vi "MarvinReport.vi"(0 "HEADER1":string="BLDC 60A CONTROLLER TEST DATA SHEET", 1 "ATR Or":refnum<vi>, 2 "Steps   pfull":string[][](table)=[["1", "Comm. & Motor Test", "", "", "", " ", ""], ["1.1", "RS232 Comm. + Version", "5.4.8", "-", "-", "", ""], ["1.2", "CAN Comm.", "5.4.8", "-", "-", "0.0.0", "FAIL"], ["1.3", "Motor Direction", "OK", "-", "-", "", ""], [" ", "", "", "", "", "", ""], ["2", "Venable Test", "", "", "", "", ""], ["2.1", "VEnable ON", "1000", "+/-100", "rpm", "", ""], ["2.2", "VEnable OFF", "0", "+/-100", "rpm", "", ""], [" ", "", "", "", "", "", ""], ["3", "Up/Down Blower Test", "", "", "", "", ""], ["3.1", "Up switch", "1000", "+/-100", "rpm", "", ""], ["3.2", "Down switch", "0", "+/-100", "rpm", "", ""], [" ", "", "", "", "", "", ""], ["4", "Resistance Merkava 4 Test", "", "", "", "", ""], ["4.1", "Resistor measure 1 position", "6850", "+/-100", "rpm", "", ""], ["4.2", "Resistor measure 2 position", "8300", "+/-100", "rpm", "", ""], ["4.3", "Resistor measure 3 position", "9200", "+/-100", "rpm", "", ""], [" ", "", "", "", "", "", ""], ["5", "Resistance Merkava 3 Test", "", "", "", "", ""], ["5.1", "Resistor measure 4 position", "6850", "+/-100", "rpm", "", ""], ["5.2", "Resistor measure 5 position", "9000", "+/-100", "rpm", "", ""], ["5.3", "Resistor measure 6 position", "9980", "+/-100", "rpm", "", ""], [" ", "", "", "", "", "", ""], ["6", "Resistance Namer Test", "", "", "", "", ""], ["6.1", "Resistor measure 7 position", "8350", "+/-100", "rpm", "", ""], ["6.2", "Resistor measure 8 position", "8900", "+/-100", "rpm", "", ""], ["6.3", "Resistor measure 9 position", "9450", "+/-100", "rpm", "", ""], [" ", "", "", "", "", "", ""], ["7", "Analog Voltage Test", "", "", "", "", ""], ["7.1", "Analog Cmd 0V (Analog Sts)", "0", "+/-0.2", "V", "", ""], ["7.2", "Analog Cmd 0V (Velocity)", "0", "+/-200", "rpm", "", ""], ["7.3", "Analog Cmd 1V (Analog Sts)", "1", "+/-0.2", "V", "", ""], ["7.4", "Analog Cmd 1V (Velocity)", "0", "+/-200", "rpm", "", ""], ["7.5", "Analog Cmd 2V (Analog Sts)", "2", "+/-0.2", "V", "", ""], ["7.6", "Analog Cmd 2V (Velocity)", "0", "+/-200", "rpm", "", ""], ["7.7", "Analog Cmd 3V (Analog Sts)", "3", "+/-0.2", "V", "", ""], ["7.8", "Analog Cmd 3V (Velocity)", "0", "+/-200", "rpm", "", ""], ["7.9", "Analog Cmd 4V (Analog Sts)", "4", "+/-0.2", "V", "", ""], ["7.10", "Analog Cmd 4V (Velocity)", "", "+/-200", "rpm", "", ""], ["7.11", "Analog Cmd 4.5V (Analog Sts)", "4.5", "+/-0.2", "V", "", ""], ["7.12", "Analog Cmd 4.5V (Velocity)", "", "+/-200", "rpm", "", ""], [" ", "", "", "", "", "", ""], ["8", "Motor Run Test", "", "", "", "", ""], ["8.1", "Motor Temperature before Run", "30", "+/-15", "C", "", ""], ["8.2", "Motor Current after 1 min", "47", "+/-3", "A", "", ""], ["8.3", "Motor Temperature after 20 min", "55", "+/-15", "C", "", ""], ["8.4", "Motor Current after 20 min", "47", "+/-3", "A", "", ""], [" ", "", "", "", "", "", ""], ["9", "Conductivity Test", "", "", "", "", ""], ["9.1", "J56 to CHASIS", "< 2m", "-", "ohms", "", ""], ["9.2", "J57 to CHASIS", "< 2m", "-", "ohms", "", ""], ["9.3", "J58 to CHASIS", "< 2m", "-", "ohms", "", ""], ["", "", "", "", "", "", ""], ["10", "Insulation Resistance Test", "", "", "", "", ""], ["10.1", "J56_A to CHASIS", "> 500k", "-", "ohms", "", ""], ["10.2", "J56_B to CHASIS", "> 500k", "-", "ohms", "", ""], ["10.3", "J56_C to CHASIS", "> 500k", "-", "ohms", "", ""], ["10.4", "J57_A to CHASIS", "> 500k", "-", "ohms", "", ""], ["10.5", "J57_B to CHASIS", "> 500k", "-", "ohms", "", ""], ["", "", "", "", "", "", ""], ["11", "Torque Test", "", "", "", "", ""], ["11.1", "Torque wrench by DIN Standard & ", "-", "-", ".", "", ""], ["11.2", "manufacturer's instructions for nut Torque.", "-", "-", ".", "", ""], ["", "", "", "", "", "", ""], ["12", "Blower Calibration", "", "", "", "", ""], ["12.1", "Motor Speed ", "9980", "+/-100", "rpm", "", ""], ["12.2", "Driver Current ", "47", "+/-3", "A", "", ""], ["", "", "", "", "", "", ""], ["13", "Leak Test", "5", "+/-0.2", "psig", "", ""], [" ", "", "", "", "", "", ""], ["14", "Set Production Parameters", "", "", "", "", ""], ["14.1", "Unit Serial number", "239", "-", "-", "", ""], [" ", "", "", "", "", "", ""]] caption="ATR", 3 "ApprovedBy":string="N_A", 5 "pageNum":i32=3, 6 "InputHeaderArray":string[][](array[string])=[["", "P/N: RD000001 ", "", "Date: 22/11/2018"], ["", "DRIVER S/N: ", "", "Time: 10:13"], ["", "Product Rev.: 2C  ", "", "Tested by: hfg"], ["", "Software Ver.: 5.4.8", "", "Approved by: GIDI"], ["", "Parameters Ver.: 0.4", "", ""], ["", "Tester Software Ver.: V0.0.o", "", ""], ["", "Tester HW Rev.: V0.1", "", ""], ["", "DSP BOARD S/N: ", "", ""], ["", "POWER BOARD S/N: ", "", ""], ["", "", "", ""], ["", "", "", ""], ["", "", "", ""], ["", "", "", ""], ["", "", "", " "]], 7 "FILE NAME":string="ATR__22-Nov-18.docx", 9 "Report Folder":path=path "C:/Users/Joseph/Desktop/KineticsReports/ATR__22-Nov-18.docx", 11 "PN":string="1", 12 "error in (no error)":errorcluster, 13 "REV":string="  Rev-5.4.8") -> (4 "path out":path=path "C:/Users/Joseph/Desktop/KineticsReports/ATR__22-Nov-18.docx", 15 "error out":errorcluster)   [LabVIEW 2017]
uses:
  <vilib>/Utility/miscctls.llb/LVRowAndColumnUnsignedTypeDef.ctl
  <vilib>/Utility/NIReport.llb/Append Image to Report (path wrap).vi
  <vilib>/Utility/NIReport.llb/Append Text Table to Report (wrap).vi
  <vilib>/Utility/NIReport.llb/Append Report Text (str wrap).vi
  <vilib>/Utility/NIReport.llb/NI_report.lvclass
  <vilib>/Utility/NIReport.llb/Word/NI_Word.lvclass
  <vilib>/addons/_office/NI_ReportGenerationToolkit.lvlib
panel:
  out "size(s)":i32[](array[numeric])
  out "error out 2":errorcluster
  out "RefArr":u32[](array[numeric])=[2875195627, 2876244204, 2878341358]
  in  "Tab Control":T1(tab)=enum."PART1 "
  out "ERRORS\nLIST":string="Summery of Results (Fails Only) :  \t1.2  FAIL !"
  out "Steps   p1":string[][](table)=[["1", "Comm. & Motor Test", "", "", "", " ", ""], ["1.1", "RS232 Comm. + Version", "5.4.8", "-", "-", "", ""], ["1.2", "CAN Comm.", "5.4.8", "-", "-", "", ""], ["1.3", "Motor Direction", "OK", "-", "-", "", ""], [" ", "", "", "", "", "", ""], ["2", "Venable Test", "", "", "", "", ""], ["2.1", "VEnable ON", "1000", "+/-100", "rpm", "", ""], ["2.2", "VEnable OFF", "0", "+/-100", "rpm", "", ""], [" ", "", "", "", "", "", ""], ["3", "Up/Down Blower Test", "", "", "", "", ""], ["3.1", "Up switch", "1000", "+/-100", "rpm", "", ""], ["3.2", "Down switch", "0", "+/-100", "rpm", "", ""], [" ", "", "", "", "", "", ""], ["4", "Resistance Merkava 4 Test", "", "", "", "", ""], ["4.1", "Resistor measure 1 position", "6850", "+/-100", "rpm", "", ""], ["4.2", "Resistor measure 2 position", "8300", "+/-100", "rpm", "", ""], ["4.3", "Resistor measure 3 position", "9200", "+/-100", "rpm", "", ""], [" ", "", "", "", "", "", ""], ["5", "Resistance Merkava 3 Test", "", "", "", "", ""], ["5.1", "Resistor measure 4 position", "6850", "+/-100", "rpm", "", ""], ["5.2", "Resistor measure 5 position", "9000", "+/-100", "rpm", "", ""], ["5.3", "Resistor measure 6 position", "9980", "+/-100", "rpm", "", ""], [" ", "", "", "", "", "", ""], ["6", "Resistance Namer Test", "", "", "", "", ""], ["6.1", "Resistor measure 7 position", "8350", "+/-100", "rpm", "", ""], ["6.2", "Resistor measure 8 position", "8900", "+/-100", "rpm", "", ""], ["6.3", "Resistor measure 9 position", "9450", "+/-100", "rpm", "", ""], [" ", "", "", "", "", "", ""], ["7", "Analog Voltage Test", "", "", "", "", ""], ["7.1", "Analog Cmd 0V (Analog Sts)", "0", "+/-0.2", "V", "", ""], ["7.2", "Analog Cmd 0V (Velocity)", "0", "+/-200", "rpm", "", ""], ["7.3", "Analog Cmd 1V (Analog Sts)", "1", "+/-0.2", "V", "", ""], ["7.4", "Analog Cmd 1V (Velocity)", "0", "+/-200", "rpm", "", ""], ["7.5", "Analog Cmd 2V (Analog Sts)", "2", "+/-0.2", "V", "", ""], ["7.6", "Analog Cmd 2V (Velocity)", "0", "+/-200", "rpm", "", ""], ["7.7", "Analog Cmd 3V (Analog Sts)", "3", "+/-0.2", "V", "", ""], ["7.8", "Analog Cmd 3V (Velocity)", "0", "+/-200", "rpm", "", ""], ["7.9", "Analog Cmd 4V (Analog Sts)", "4", "+/-0.2", "V", "", ""], ["7.10", "Analog Cmd 4V (Velocity)", "", "+/-200", "rpm", "", ""], ["7.11", "Analog Cmd 4.5V (Analog Sts)", "4.5", "+/-0.2", "V", "", ""], ["7.12", "Analog Cmd 4.5V (Velocity)", "", "+/-200", "rpm", "", ""], [" ", "", "", "", "", "", ""], ["8", "Motor Run Test", "", "", "", "", ""], ["8.1", "Motor Temperature before Run", "30", "+/-15", "C", "", ""], ["8.2", "Motor Current after 1 min", "47", "+/-3", "A", "", ""], ["8.3", "Motor Temperature after 20 min", "55", "+/-15", "C", "", ""], ["8.4", "Motor Current after 20 min", "47", "+/-3", "A", "", ""], [" ", "", "", "", "", "", ""], ["9", "Conductivity Test", "", "", "", "", ""], ["9.1", "J56 to CHASIS", "< 2m", "-", "ohms", "", ""], ["9.2", "J57 to CHASIS", "< 2m", "-", "ohms", "", ""], ["9.3", "J58 to CHASIS", "< 2m", "-", "ohms", "", ""], ["", "", "", "", "", "", ""], ["10", "Insulation Resistance Test", "", "", "", "", ""], ["10.1", "J56_A to CHASIS", "> 500k", "-", "ohms", "", ""], ["10.2", "J56_B to CHASIS", "> 500k", "-", "ohms", "", ""], ["10.3", "J56_C to CHASIS", "> 500k", "-", "ohms", "", ""], ["10.4", "J57_A to CHASIS", "> 500k", "-", "ohms", "", ""], ["10.5", "J57_B to CHASIS", "> 500k", "-", "ohms", "", ""], ["", "", "", "", "", "", ""], ["11", "Torque Test", "", "", "", "", ""], ["11.1", "Torque wrench by DIN Standard & ", "-", "-", ".", "", ""], ["11.2", "manufacturer's instructions for nut Torque.", "-", "-", ".", "", ""], ["", "", "", "", "", "", ""], ["12", "Blower Calibration", "", "", "", "", ""], ["12.1", "Motor Speed ", "9980", "+/-100", "rpm", "", ""], ["12.2", "Driver Current ", "47", "+/-3", "A", "", ""], ["", "", "", "", "", "", ""], ["13", "Leak Test", "5", "+/-0.2", "psig", "", ""], [" ", "", "", "", "", "", ""], ["14", "Set Production Parameters", "", "", "", "", ""], ["14.1", "Unit Serial number", "239", "-", "-", "", ""], [" ", "", "", "", "", "", ""]] caption="ATR"
  out "Steps   p2":string[][](table)=[["1", "Comm. & Motor Test", "", "", "", " ", ""], ["1.1", "RS232 Comm. + Version", "5.4.8", "-", "-", "", ""], ["1.2", "CAN Comm.", "5.4.8", "-", "-", "0.0.0", "FAIL"], ["1.3", "Motor Direction", "OK", "-", "-", "", ""], [" ", "", "", "", "", "", ""], ["2", "Venable Test", "", "", "", "", ""], ["2.1", "VEnable ON", "1000", "+/-100", "rpm", "", ""], ["2.2", "VEnable OFF", "0", "+/-100", "rpm", "", ""], [" ", "", "", "", "", "", ""], ["3", "Up/Down Blower Test", "", "", "", "", ""], ["3.1", "Up switch", "1000", "+/-100", "rpm", "", ""], ["3.2", "Down switch", "0", "+/-100", "rpm", "", ""], [" ", "", "", "", "", "", ""], ["4", "Resistance Merkava 4 Test", "", "", "", "", ""], ["4.1", "Resistor measure 1 position", "6850", "+/-100", "rpm", "", ""], ["4.2", "Resistor measure 2 position", "8300", "+/-100", "rpm", "", ""], ["4.3", "Resistor measure 3 position", "9200", "+/-100", "rpm", "", ""], [" ", "", "", "", "", "", ""], ["5", "Resistance Merkava 3 Test", "", "", "", "", ""], ["5.1", "Resistor measure 4 position", "6850", "+/-100", "rpm", "", ""], ["5.2", "Resistor measure 5 position", "9000", "+/-100", "rpm", "", ""], ["5.3", "Resistor measure 6 position", "9980", "+/-100", "rpm", "", ""], [" ", "", "", "", "", "", ""], ["6", "Resistance Namer Test", "", "", "", "", ""], ["6.1", "Resistor measure 7 position", "8350", "+/-100", "rpm", "", ""], ["6.2", "Resistor measure 8 position", "8900", "+/-100", "rpm", "", ""], ["6.3", "Resistor measure 9 position", "9450", "+/-100", "rpm", "", ""], [" ", "", "", "", "", "", ""], ["7", "Analog Voltage Test", "", "", "", "", ""], ["7.1", "Analog Cmd 0V (Analog Sts)", "0", "+/-0.2", "V", "", ""], ["7.2", "Analog Cmd 0V (Velocity)", "0", "+/-200", "rpm", "", ""], ["7.3", "Analog Cmd 1V (Analog Sts)", "1", "+/-0.2", "V", "", ""], ["7.4", "Analog Cmd 1V (Velocity)", "0", "+/-200", "rpm", "", ""], ["7.5", "Analog Cmd 2V (Analog Sts)", "2", "+/-0.2", "V", "", ""], ["7.6", "Analog Cmd 2V (Velocity)", "0", "+/-200", "rpm", "", ""], ["7.7", "Analog Cmd 3V (Analog Sts)", "3", "+/-0.2", "V", "", ""], ["7.8", "Analog Cmd 3V (Velocity)", "0", "+/-200", "rpm", "", ""], ["7.9", "Analog Cmd 4V (Analog Sts)", "4", "+/-0.2", "V", "", ""], ["7.10", "Analog Cmd 4V (Velocity)", "", "+/-200", "rpm", "", ""], ["7.11", "Analog Cmd 4.5V (Analog Sts)", "4.5", "+/-0.2", "V", "", ""], ["7.12", "Analog Cmd 4.5V (Velocity)", "", "+/-200", "rpm", "", ""], [" ", "", "", "", "", "", ""], ["8", "Motor Run Test", "", "", "", "", ""], ["8.1", "Motor Temperature before Run", "30", "+/-15", "C", "", ""], ["8.2", "Motor Current after 1 min", "47", "+/-3", "A", "", ""], ["8.3", "Motor Temperature after 20 min", "55", "+/-15", "C", "", ""], ["8.4", "Motor Current after 20 min", "47", "+/-3", "A", "", ""], [" ", "", "", "", "", "", ""], ["9", "Conductivity Test", "", "", "", "", ""], ["9.1", "J56 to CHASIS", "< 2m", "-", "ohms", "", ""], ["9.2", "J57 to CHASIS", "< 2m", "-", "ohms", "", ""], ["9.3", "J58 to CHASIS", "< 2m", "-", "ohms", "", ""], ["", "", "", "", "", "", ""], ["10", "Insulation Resistance Test", "", "", "", "", ""], ["10.1", "J56_A to CHASIS", "> 500k", "-", "ohms", "", ""], ["10.2", "J56_B to CHASIS", "> 500k", "-", "ohms", "", ""], ["10.3", "J56_C to CHASIS", "> 500k", "-", "ohms", "", ""], ["10.4", "J57_A to CHASIS", "> 500k", "-", "ohms", "", ""], ["10.5", "J57_B to CHASIS", "> 500k", "-", "ohms", "", ""], ["", "", "", "", "", "", ""], ["11", "Torque Test", "", "", "", "", ""], ["11.1", "Torque wrench by DIN Standard & ", "-", "-", ".", "", ""], ["11.2", "manufacturer's instructions for nut Torque.", "-", "-", ".", "", ""], ["", "", "", "", "", "", ""], ["12", "Blower Calibration", "", "", "", "", ""], ["12.1", "Motor Speed ", "9980", "+/-100", "rpm", "", ""], ["12.2", "Driver Current ", "47", "+/-3", "A", "", ""], ["", "", "", "", "", "", ""], ["13", "Leak Test", "5", "+/-0.2", "psig", "", ""], [" ", "", "", "", "", "", ""], ["14", "Set Production Parameters", "", "", "", "", ""], ["14.1", "Unit Serial number", "239", "-", "-", "", ""], [" ", "", "", "", "", "", ""]] caption="ATR"
  in  "Fail  Button":bool
  in  "Pass  Button":bool
  # "e"
  # "e"
  # "<pre>"
  # "for html"
  # "for html"
  # "</pre>"
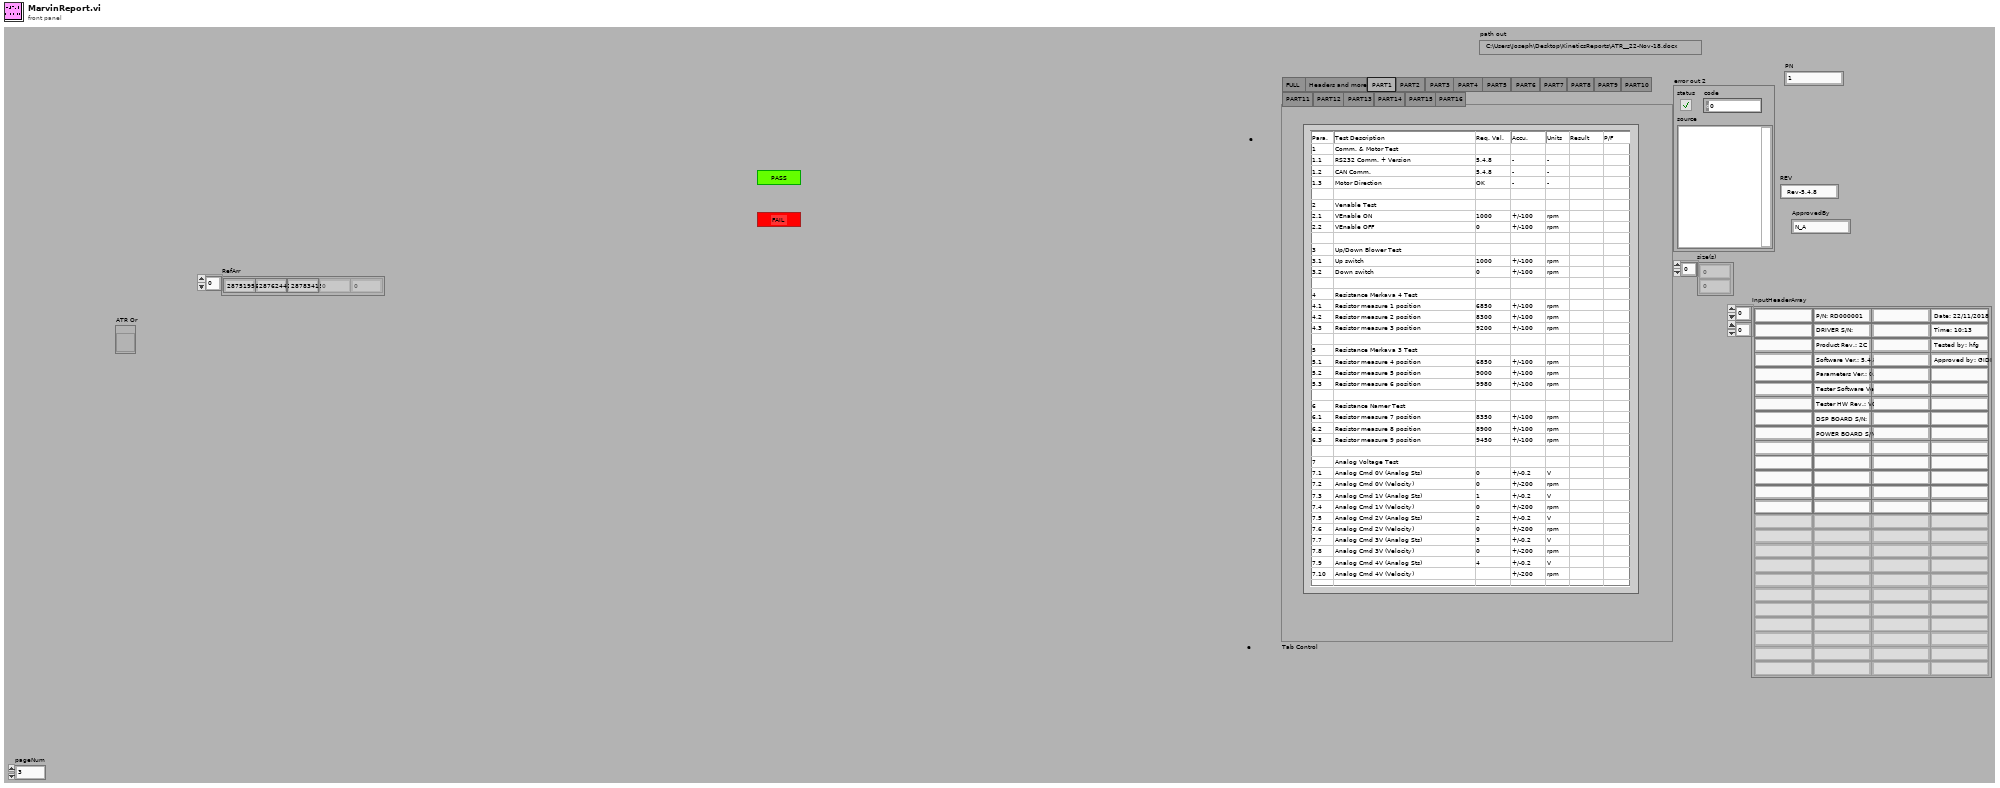
[diagram p1: front panel]
types:
  T1 = enum32{"FULL", "Headers and more", "PART1 ", "PART2 ", "PART3 ", "PART4 ", "PART5 ", "PART6 ", "PART7", "PART8", "PART9", "PART10", "PART11", "PART12", "PART13", "PART14", "PART15", "PART16"}
  T2 = typedef "LVRowAndColumnUnsignedTypeDef.ctl" = cluster{"Row":u32, "Column":u32}
  T3 = cluster{"position (excel)":cluster{"row":i32, "column":i32}, "name (excel)":string, "bookmark (word)":string}
  T4 = cluster{"top":dbl, "left":dbl, "right":dbl, "bottom":dbl}
  T5 = enum16{"Standard Report", "HTML", "Word", "Excel"}
  T6 = cluster{"Italic":enum16{"Italic Unchanged", "Italic On", "Italic Off"}, "Strike Through":enum16{"Strike Through Unchanged", "Strike Through On", "Strike Through Off"}, "Underline":enum16{"Underline Unchanged", "Underline On", "Underline Off"}, "Bold":enum16{"Bold Unchanged", "Bold On", "Bold Off"}}
  T7 = cluster{"charset (-1)":i16, "weight (-1)":i16, "name":string, "size":string}
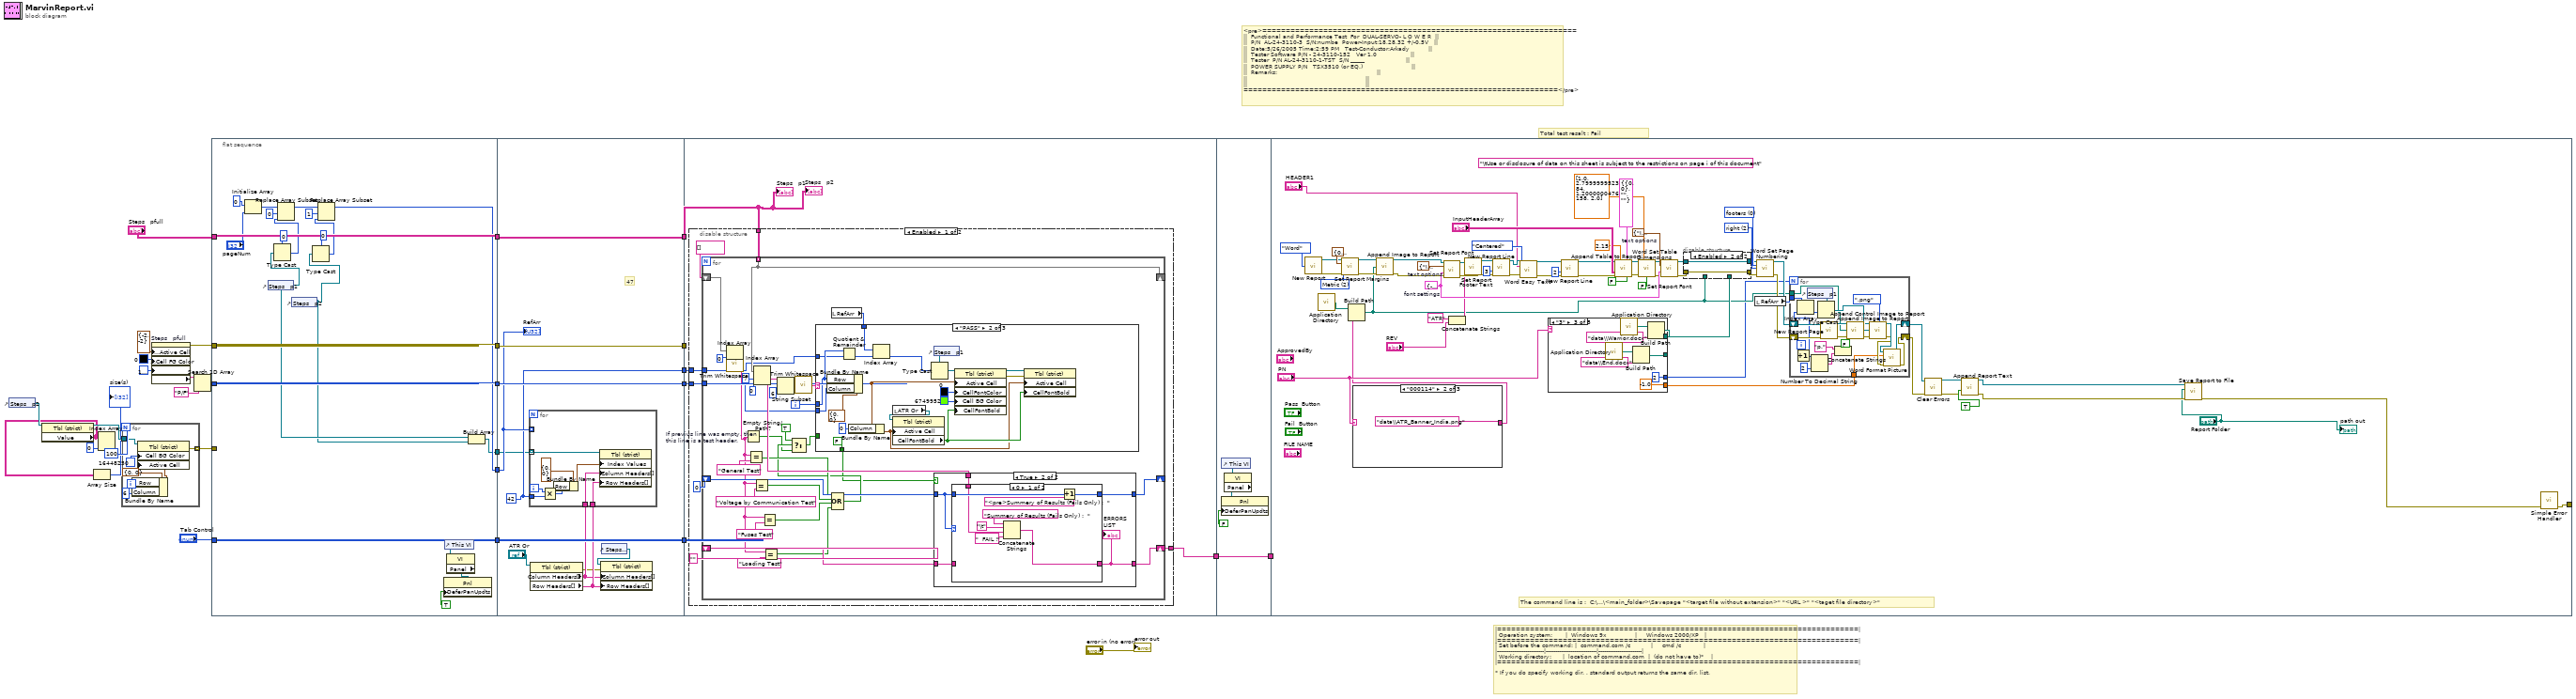
[diagram p0: block diagram]
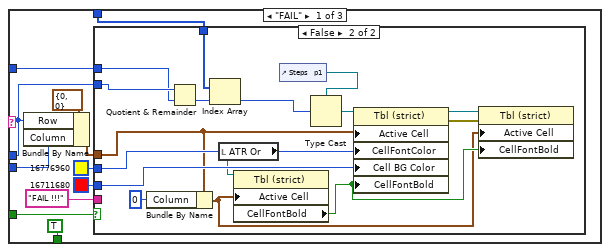
[diagram p2: hidden frame]
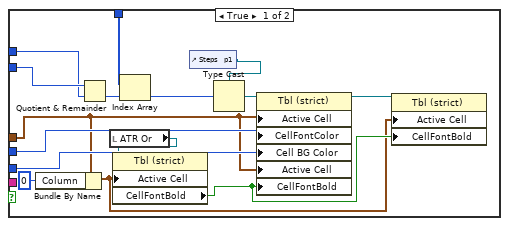
[diagram p3: hidden frame]
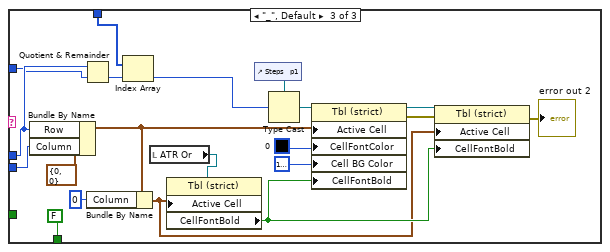
[diagram p4: hidden frame]
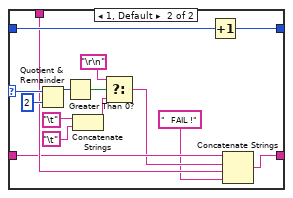
[diagram p6: hidden frame]
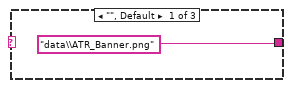
[diagram p8: hidden frame]
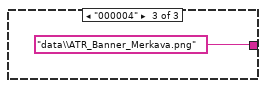
[diagram p9: hidden frame]
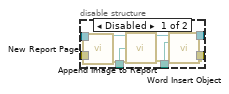
[diagram p10: hidden frame]
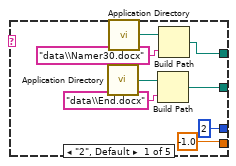
[diagram p11: hidden frame]
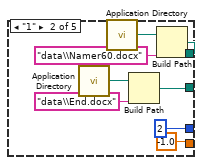
[diagram p12: hidden frame]
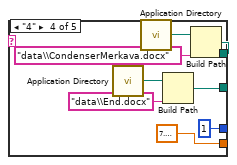
[diagram p13: hidden frame]
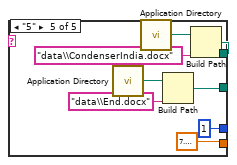
[diagram p14: hidden frame]
diagram:
  # "Total test resalt : Fail"
  # "|=============================================================================|\n| Operation system:       |  Windows 9x               |     Windows 2000/XP   |\n|=============================================================================|\n| Set before the command: |  command.com /c           |     cmd /c            |\n|-------------------------|---------------------------|-----------------------|\n| Working directory:      |  location of command.com  |  (do not have to)*    |\n|=============================================================================|\n\n* If you do specify working dir. , standard output returns the same dir. list."
  # "<pre>===================================================================\n||  Functional and Performance Test  For  DUAL-SERVO- L O W E R  ||\n||  P/N  AL-24-3110-3  S/N:numbe  Power-Input:18,28,32 +/-0.5V   ||\n||  Date:5/26/2005 Time:2:59 PM   Test-Conductor:Arkady          ||\n||  Tester Software P/N - 24-3110-152   Ver 1.0                  ||\n||  Tester  P/N AL-24-3110-1-TST  S/N _____                      ||\n||  POWER SUPPLY P/N   TSX3510 (or EQ.)                          ||\n||  Remarks:                                                     ||\n||                                                               ||\n||                                                               ||\n===================================================================</pre>"
  n1 = control-ref of="Steps   p2"() -> (w4:refnum<vi>)
  n2 = property class="Tbl (strict)"(reference=w4) -> ("Value"=w2:string[][])  [unwired: 1 in, 2 out]
  n3 = Array Size(array=w2) -> (size(s)=→"size(s)":i32[])
  n4 = Index Array(array=w2, index (col)=0 ("disabled index (col)")) -> ()  [unwired: 1 in, 1 out]
  n5 = for {
    N: 100 -> [_]
    tunnel: w4 -> [w36]
    tunnel: [w31] -> w5 mode=indexing
    i -> [w32]
    n6 = Bundle By Name(cluster=cluster{"Row":i32, "Column":i32} {"Row"=0, "Column"=0} ("Active Cell"), "Row"=w32, "Column"=6) -> (w33:cluster{"Row":i32, "Column":i32})
    n7 = property class="Tbl (strict)"(reference=w36, "Cell BG Color"=u32 16448250, "Active Cell"=w33) -> (error out=w31:errorcluster)  [unwired: 1 in, 1 out]
  }
  n8 = property on="Steps   pfull" class="Tbl (strict)"("Active Cell:Active Cell"=cluster{"Row":i32, "Column":i32} {"Row"=-2, "Column"=-2} ("Active Cell"), "Active Cell:Cell FG Color"=u32 0, "Active Cell:Cell Background Color"=u32 16777226) -> (error out=w26:errorcluster, "Column Header Strings[]"=w24:string[])  [unwired: 2 in, 1 out]
  n9 = Search 1D Array(1D array=w24, element="P/F") -> (index of element=w23:i32)  [unwired: 1 in]
  n10 = flat-sequence {
    tunnel: "Tab Control" -> [w54]
    tunnel: w23 -> [w55]
    tunnel: w26 -> [w56]
    tunnel: "Steps   pfull" -> [w57]
    tunnel: [w57] -> w15
    tunnel: [w56] -> w14
    tunnel: [w55] -> w13
    tunnel: [w54] -> w12
    tunnel: [w50] -> w9
    tunnel: [w37] -> w7
    tunnel: w5 -> [_]
    tunnel: [w69] -> w19
    tunnel: [w68] -> w18
    tunnel: [w67] -> w17
    tunnel: [w66] -> w16
    tunnel: w15 -> [w69]
    tunnel: w14 -> [w68]
    tunnel: w13 -> [w67]
    tunnel: w12 -> [w66]
    tunnel: w9 -> [w65]
    tunnel: [w64] -> w8
    tunnel: w7 -> [w58]
    tunnel: [w80] -> w11
    tunnel: w19 -> [w78]
    tunnel: w18 -> [_]
    tunnel: w17 -> [w81]
    tunnel: w16 -> [_]
    tunnel: w8 -> [w79]
    tunnel: w11 -> [w235]
    tunnel: [w235] -> w10
    tunnel: [w298] -> _
    tunnel: w10 -> [_]
    frame #0 {
      n11 = Initialize Array "Initialize Array"(u32 0, "pageNum") -> (w43:u32[])
      n12 = control-ref of="Steps   p1"() -> (w39:refnum<vi>)
      n13 = Type Cast(type=u32 0, x=w39) -> (*(type *) &x=w44:u32)
      n14 = Replace Array Subset(array=w43, new element=w44, index=0) -> (w47:u32[])
      n15 = control-ref of="Steps   p2"() -> (w38:refnum<vi>)
      n16 = Type Cast(type=u32 0, x=w38) -> (*(type *) &x=w48:u32)
      n17 = Replace Array Subset(array=w47, new element=w48, index=1) -> (w50:u32[])
      n18 = control-ref of="This VI"() -> (w51:refnum<vi>)
      n19 = property class="VI"(reference=w51) -> ("Panel"=w52:refnum<vi>)  [unwired: 1 in, 2 out]
      n20 = property class="Pnl"(reference=w52, "DeferPanUpdts"=TRUE ("Defer Panel Updates")) -> ()  [unwired: 1 in, 2 out]
      n21 = Build Array(w39, w38) -> (w37:refnum<vi>[])
    }
    frame #1 {
      w64 = u32 42 ("Row")
      # "47"
      n22 = property class="Tbl (strict)"(reference="ATR Or") -> (error out=w61:errorcluster, "Column Headers[]"=w62:string[], "Row Headers[]"=w63:string[])  [unwired: 1 in, 1 out]
      n23 = for {
        tunnel: w65 -> [_] mode=indexing
        tunnel: w62 -> [w73]
        tunnel: w63 -> [w72]
        tunnel: w64 -> [w71]
        tunnel: w58 -> [w70] mode=indexing
        i -> [w75]
        n24 = Multiply(x=w75, y=w71) -> (x*y=w74:u32)
        n25 = Bundle By Name(cluster=T2 {"Row"=0, "Column"=0} ("Index Values"), "Row"=w74) -> (w76:T2)
        n26 = property class="Tbl (strict)"(reference=w70, "Index Values"=w76, "Column Headers[]"=w73, "Row Headers[]"=w72) -> ()  [unwired: 1 in, 2 out]
      }
      n27 = control-ref of="Steps   pfull"() -> (w59:refnum<vi>)
      n28 = property class="Tbl (strict)"(reference=w59, error in=w61, "Column Headers[]"=w62, "Row Headers[]"=w63) -> ()  [unwired: 2 out]
      "RefArr" <- w65
    }
    frame #2 {
      n29 = disable-structure shown="Enabled" {
        disable-tunnel: w81 -> [w88 _]
        disable-tunnel: [w87 _] -> w80
        disable-tunnel: w78 -> [w83 _]
        disable-tunnel: w79 -> [w82 _]
        frame Enabled {
          n30 = for {
            tunnel: w83 -> [w120] mode=indexing
            shift-right: [w120] -> _
            shift-left: string[] [] ("ATR in") -> [w119]
            tunnel: w88 -> [w96]
            shift-right: [w111] -> w87
            shift-left: "" ("trimmed string") -> [w115]
            shift-right: [w114] -> _
            shift-left: 0 -> [w113]
            tunnel: w82 -> [w92]
            i -> [w97]
            n31 = Index Array(array=w119, index=0) -> (element=w117:string)
            n32 = call <vilib>:"Trim Whitespace.vi"("string"=w117) -> ("trimmed string"=w93:string)  [unwired: 1 in]
            n33 = Empty String/Path? "If previus line was empty, then\nthis line is a test header."(string/path=w93) -> (empty?=w99:bool)
            n34 = Equal?(x=w93, y="General Test") -> (x = y?=w108:bool)
            n35 = Equal?(x=w93, y="Voltage by Communication Test") -> (x = y?=w103:bool)
            n36 = Index Array(array=w120, index #1=7 ("index"), index #2=0) -> (element #1=w116:string, element #2=w112:string)
            n37 = Equal?(x=w93, y="Fuses Test") -> (x = y?=w104:bool)
            n38 = Equal?(x=w93, y="Loading Test") -> (x = y?=w105:bool)
            n39 = String Subset(string=w116, length (rest)=6 ("length (rest)")) -> (substring=w121:string)  [unwired: 1 in]
            n40 = call <vilib>:"Trim Whitespace.vi"("string"=w121) -> ("trimmed string"=w98:string)  [unwired: 1 in]
            n41 = local read "RefArr"() -> (w89:u32[])
            n42 = Compound Arithmetic op=OR(w108, w103, w104, w105) -> (w106:bool)
            n43 = Select(t=TRUE, s=w106, f=w99) -> (s? t:f=w95:bool)
            n44 = case shown="\"PASS\"" w98 {
              tunnel: w97 -> [w124 w177 w198]
              tunnel: w96 -> [w126 w181 w201]
              tunnel: w95 -> [w128 _ _]
              tunnel: [TRUE FALSE FALSE] -> w94
              tunnel: w89 -> [w125 w175 w197]
              tunnel: w92 -> [w122 w164 w183]
              frame "FAIL" {
                n45 = Bundle By Name(cluster=cluster{"Row":i32, "Column":i32} {"Row"=0, "Column"=0} ("Active Cell"), "Row"=w124, "Column"=w126) -> (w132:cluster{"Row":i32, "Column":i32})
                n46 = case shown="False" w128 {
                  tunnel: w132 -> [w140 w152]
                  tunnel: u32 16776960 -> [w147 w163]
                  tunnel: u32 16711680 -> [w146 w162]
                  tunnel: "FAIL !!!" ("string") -> [_ _]
                  tunnel: w125 -> [w144 w159]
                  tunnel: w124 -> [w143 w160]
                  tunnel: w122 -> [w133 w148]
                  frame True {
                    n47 = Bundle By Name(cluster=w140, "Column"=0) -> (w136:cluster{"Row":i32, "Column":i32})
                    n48 = Quotient & Remainder(x=w143, y=w133) -> (floor(x/y)=w145:u32)  [unwired: 1 out]
                    n49 = local read "ATR Or"() -> (w134:refnum<vi>)
                    n50 = property class="Tbl (strict)"(reference=w134, "Active Cell"=w136) -> ("CellFontBold"=w137:bool)  [unwired: 1 in, 2 out]
                    n51 = Index Array(array=w144, index=w145) -> (element=w141:u32)
                    n52 = control-ref of="Steps   p1"() -> (w135:refnum<vi>)
                    n53 = Type Cast(type=w135, x=w141) -> (*(type *) &x=w142:refnum<vi>)
                    n54 = property class="Tbl (strict)"(reference=w142, "Active Cell"=w140, "CellFontColor"=w147, "Cell BG Color"=w146, "Active Cell"=w140, "CellFontBold"=w137) -> (reference out=w138:refnum<vi>)  [unwired: 1 in, 1 out]
                    n55 = property class="Tbl (strict)"(reference=w138, "Active Cell"=w136, "CellFontBold"=w137) -> ()  [unwired: 1 in, 2 out]
                  }
                  frame False {
                    n56 = Bundle By Name(cluster=w152, "Column"=0) -> (w151:cluster{"Row":i32, "Column":i32})
                    n57 = Quotient & Remainder(x=w160, y=w148) -> (floor(x/y)=w161:u32)  [unwired: 1 out]
                    n58 = Index Array(array=w159, index=w161) -> (element=w158:u32)
                    n59 = local read "ATR Or"() -> (w150:refnum<vi>)
                    n60 = property class="Tbl (strict)"(reference=w150, "Active Cell"=w151) -> ("CellFontBold"=w154:bool)  [unwired: 1 in, 2 out]
                    n61 = control-ref of="Steps   p1"() -> (w149:refnum<vi>)
                    n62 = Type Cast(type=w149, x=w158) -> (*(type *) &x=w157:refnum<vi>)
                    n63 = property class="Tbl (strict)"(reference=w157, "Active Cell"=w152, "CellFontColor"=w163, "Cell BG Color"=w162, "CellFontBold"=w154) -> (reference out=w156:refnum<vi>, error out=w155:errorcluster)  [unwired: 1 in]
                    n64 = property class="Tbl (strict)"(reference=w156, error in=w155, "Active Cell"=w151, "CellFontBold"=w154) -> ()  [unwired: 2 out]
                  }
                }
              }
              frame "PASS" {
                n65 = Bundle By Name(cluster=cluster{"Row":i32, "Column":i32} {"Row"=0, "Column"=0} ("Active Cell"), "Row"=w177, "Column"=w181) -> (w168:cluster{"Row":i32, "Column":i32})
                n66 = Quotient & Remainder(x=w177, y=w164) -> (floor(x/y)=w176:u32)  [unwired: 1 out]
                n67 = Bundle By Name(cluster=w168, "Column"=0) -> (w167:cluster{"Row":i32, "Column":i32})
                n68 = Index Array(array=w175, index=w176) -> (element=w174:u32)
                n69 = local read "ATR Or"() -> (w165:refnum<vi>)
                n70 = property class="Tbl (strict)"(reference=w165, "Active Cell"=w167) -> ("CellFontBold"=w170:bool)  [unwired: 1 in, 2 out]
                n71 = control-ref of="Steps   p1"() -> (w166:refnum<vi>)
                n72 = Type Cast(type=w166, x=w174) -> (*(type *) &x=w173:refnum<vi>)
                n73 = property class="Tbl (strict)"(reference=w173, "Active Cell"=w168, "CellFontColor"=u32 0, "Cell BG Color"=u32 6749952, "CellFontBold"=w170) -> (reference out=w171:refnum<vi>, error out=w172:errorcluster)  [unwired: 1 in]
                n74 = property class="Tbl (strict)"(reference=w171, error in=w172, "Active Cell"=w167, "CellFontBold"=w170) -> ()  [unwired: 2 out]
              }
              frame "_", Default {
                n75 = Bundle By Name(cluster=cluster{"Row":i32, "Column":i32} {"Row"=0, "Column"=0} ("Active Cell"), "Row"=w198, "Column"=w201) -> (w191:cluster{"Row":i32, "Column":i32})
                n76 = Quotient & Remainder(x=w198, y=w183) -> (floor(x/y)=w199:u32)  [unwired: 1 out]
                n77 = Bundle By Name(cluster=w191, "Column"=0) -> (w187:cluster{"Row":i32, "Column":i32})
                n78 = Index Array(array=w197, index=w199) -> (element=w196:u32)
                n79 = local read "ATR Or"() -> (w185:refnum<vi>)
                n80 = property class="Tbl (strict)"(reference=w185, "Active Cell"=w187) -> ("CellFontBold"=w188:bool)  [unwired: 1 in, 2 out]
                n81 = control-ref of="Steps   p1"() -> (w186:refnum<vi>)
                n82 = Type Cast(type=w186, x=w196) -> (*(type *) &x=w193:refnum<vi>)
                n83 = property class="Tbl (strict)"(reference=w193, "Active Cell"=w191, "CellFontColor"=u32 0, "Cell BG Color"=u32 16777226, "CellFontBold"=w188) -> (reference out=w190:refnum<vi>, error out=w189:errorcluster)  [unwired: 1 in]
                n84 = property class="Tbl (strict)"(reference=w190, error in=w189, "Active Cell"=w187, "CellFontBold"=w188) -> (error out=→"error out 2":errorcluster)  [unwired: 1 out]
              }
            }
            n85 = case shown="True" w94 {
              tunnel: w115 -> [w204 w206]
              tunnel: [w204 w205] -> w111
              tunnel: w113 -> [w203 w208]
              tunnel: [w203 w209] -> w114
              tunnel: w112 -> [_ w207]
              frame False {
              }
              frame True {
                n86 = case shown="0" w208 {
                  selector: w208 -> [_ w230]
                  tunnel: [w211 w220] -> w209
                  tunnel: w208 -> [w216 w231]
                  tunnel: w207 -> [w215 w227]
                  tunnel: [w213 w226] -> w205
                  tunnel: w206 -> [_ w225]
                  frame 0 {
                    (unwired) "<pre>Summery of Results (Fails Only) :  "
                    n87 = Concatenate Strings("Summery of Results (Fails Only) :  ", "\t", w215, "  FAIL !" ("string")) -> (w213:string)
                    n88 = Increment(x=w216) -> (x+1=w211:i32)
                  }
                  frame 1, Default {
                    n89 = Quotient & Remainder(x=w230, y=2) -> (x-y*floor(x/y)=w228:i32)  [unwired: 1 out]
                    n90 = Greater Than 0?(x=w228) -> (x > 0?=w224:bool)
                    n91 = Concatenate Strings("\t", "\t") -> (w219:string)
                    n92 = Select(t="\r\n", s=w224, f=w219) -> (s? t:f=w222:string)
                    n93 = Increment(x=w231) -> (x+1=w220:i32)
                    n94 = Concatenate Strings(w225, w222, w227, "  FAIL !" ("string")) -> (w226:string)
                  }
                }
                "ERRORS\nLIST" <- w205
              }
            }
          }
        }
        frame Disabled {
        }
      }
      "Steps   p1" <- w78
      "Steps   p2" <- w78
    }
    frame #3 {
      n95 = control-ref of="This VI"() -> (w232:refnum<vi>)
      n96 = property class="VI"(reference=w232) -> ("Panel"=w233:refnum<vi>)  [unwired: 1 in, 2 out]
      n97 = property class="Pnl"(reference=w233, "DeferPanUpdts"=FALSE ("Defer Panel Updates")) -> ()  [unwired: 1 in, 2 out]
    }
    frame #4 {
      w279 = u16 2 items=["Default", "US", "Metric"] ("measurement system (default)")
      (unwired) "\tUse or disclosure of data on this sheet is subject to the restrictions on page i of this document" ("center footer text")
      w286 = u16 2 items=["left", "center", "right"] ("alignment (right)")
      w287 = u16 0 items=["footers", "headers"] ("position (footers)")
      w296 = T6 {"Italic"=enum."Italic Off", "Strike Through"=enum."Strike Through Off", "Underline"=enum."Underline Off", "Bold"=enum."Bold Off"}  # text options
      w299 = T6 {"Italic"=enum."Italic Off", "Strike Through"=enum."Strike Through Off", "Underline"=enum."Underline Off", "Bold"=enum."Bold Off"}  # text options
      w297 = T7 {"charset (-1)"=-1, "weight (-1)"=-1, "name"="Tahoma", "size"="12"}  # font settings
      # "The command line is :  C:\\...\\<main_folder>\\Savepage \"<target file without extension>\" \"<URL >\" \"<taget file directory>\""
      n98 = call <vilib>:"New Report.vi"("report type"=T5."Word") -> ("report out"=w277:refnum<class "NI_report.lvclass">, "error out"=w278:errorcluster)  [unwired: 13 in]
      n99 = call <vilib>:"Application Directory.vi"() -> ("Application Directory"=w272:path)
      n100 = call-dynamic "Set Report Margins.vi"("report in"=w277, "margins (1.00)"=T4 {"top"=0.1, "left"=2.0, "right"=1.0, "bottom"=0.75}, "measurement system (default)"=w279, "error in (no error)"=w278) -> ("report out"=w276:refnum<class "NI_report.lvclass">, "error out"=w275:errorcluster)  [unwired: 9 in, 1 out]
      n101 = case shown="\"000114\"" "PN" {
        tunnel: ["data\\ATR_Banner.png" ("name or relative path") "data\\ATR_Banner_India.png" ("name or relative path") "data\\ATR_Banner_Merkava.png" ("name or relative path")] -> w236
        frame "", Default {
        }
        frame "000114" {
        }
        frame "000004" {
        }
      }
      n102 = Build Path(base path=w272, name or relative path=w236) -> (appended path=w244:path)
      n103 = call-poly <vilib>:"Append Image to Report.vi"("report in"=w276, "path or URL of image"=w244, "error in (no error)"=w275) -> ("report out"=w273:refnum<class "NI_report.lvclass">, "error out"=w274:errorcluster)  [unwired: 9 in, 2 out]
      n104 = call-dynamic "Set Report Font.vi"("report in"=w273, "text options"=w299, "font settings"=w297, "error in (no error)"=w274) -> ("report out"=w295:refnum<class "NI_report.lvclass">, "error out"=w292:errorcluster)  [unwired: 9 in, 1 out]
      n105 = Concatenate Strings("ATR" ("string"), "REV") -> (w281:string)
      n106 = call-dynamic "Set Report Footer Text.vi"("report in"=w295, "left footer text"=w281, "error in (no error)"=w292) -> ("report out"=w294:refnum<class "NI_report.lvclass">, "error out"=w293:errorcluster)  [unwired: 11 in]
      n107 = call-dynamic "New Report Line.vi"("report in"=w294, "number of lines (1)"=3, "error in (no error)"=w293) -> ("report out"=w267:refnum<class "NI_report.lvclass">, "error out"=w266:errorcluster)  [unwired: 11 in]
      n108 = call <vilib>:"Word Easy Text.vi"("report in"=w267, "text"="HEADER1", "alignment (left)"=enum16{"Left", "Centered", "Right", "Justify"}."Centered", "error in (no error)"=w266) -> ("report out"=w253:refnum<class "NI_report.lvclass">, "error out"=w254:errorcluster)  [unwired: 9 in, 1 out]
      n109 = case shown="\"3\"" "PN" {
        tunnel: [w320 w328 w336 w344 w352] -> w247
        tunnel: [w317 w325 w333 w341 w349] -> _
        tunnel: [2 2 2 1 1] -> w241
        tunnel: [sgl -1.0 ("height (-1)") sgl -1.0 ("height (-1)") sgl -1.0 ("height (-1)") sgl 7.7 ("height (-1)") sgl 7.7 ("height (-1)")] -> w239
        frame "2", Default {
          n110 = call <vilib>:"Application Directory.vi"() -> ("Application Directory"=w318:path)
          n111 = call <vilib>:"Application Directory.vi"() -> ("Application Directory"=w322:path)
          n112 = Build Path(base path=w318, name or relative path="data\\End.docx") -> (appended path=w317:path)
          n113 = Build Path(base path=w322, name or relative path="data\\Namer30.docx") -> (appended path=w320:path)
        }
        frame "1" {
          n114 = call <vilib>:"Application Directory.vi"() -> ("Application Directory"=w326:path)
          n115 = call <vilib>:"Application Directory.vi"() -> ("Application Directory"=w330:path)
          n116 = Build Path(base path=w326, name or relative path="data\\End.docx") -> (appended path=w325:path)
          n117 = Build Path(base path=w330, name or relative path="data\\Namer60.docx") -> (appended path=w328:path)
        }
        frame "3" {
          n118 = call <vilib>:"Application Directory.vi"() -> ("Application Directory"=w334:path)
          n119 = call <vilib>:"Application Directory.vi"() -> ("Application Directory"=w338:path)
          n120 = Build Path(base path=w334, name or relative path="data\\End.docx") -> (appended path=w333:path)
          n121 = Build Path(base path=w338, name or relative path="data\\Warrior.docx") -> (appended path=w336:path)
        }
        frame "4" {
          n122 = call <vilib>:"Application Directory.vi"() -> ("Application Directory"=w342:path)
          n123 = call <vilib>:"Application Directory.vi"() -> ("Application Directory"=w346:path)
          n124 = Build Path(base path=w342, name or relative path="data\\End.docx") -> (appended path=w341:path)
          n125 = Build Path(base path=w346, name or relative path="data\\CondenserMerkava.docx") -> (appended path=w344:path)
        }
        frame "5" {
          n126 = call <vilib>:"Application Directory.vi"() -> ("Application Directory"=w350:path)
          n127 = call <vilib>:"Application Directory.vi"() -> ("Application Directory"=w354:path)
          n128 = Build Path(base path=w350, name or relative path="data\\End.docx") -> (appended path=w349:path)
          n129 = Build Path(base path=w354, name or relative path="data\\CondenserIndia.docx") -> (appended path=w352:path)
        }
      }
      n130 = call-dynamic "New Report Line.vi"("report in"=w253, "number of lines (1)"=2, "error in (no error)"=w254) -> ("report out"=w252:refnum<class "NI_report.lvclass">, "error out"=w251:errorcluster)  [unwired: 11 in]
      n131 = call-poly <vilib>:"Append Table to Report.vi"("report in"=w252, "column width (1)"=2.15, "MS Office parameters"=T3 {"position (excel)"={"row"=0, "column"=0}, "name (excel)"="", "bookmark (word)"=""}, "text data"="InputHeaderArray", "error in (no error)"=w251, "show grid lines (YES)"=FALSE) -> ("report out"=w259:refnum<class "NI_report.lvclass">, "error out"=w258:errorcluster)  [unwired: 6 in, 2 out]
      n132 = call <vilib>:"Word Set Table Dimensions.vi"("report in"=w259, "table column widths"=sgl[] [1.0, 2.8, 1.2, 2.0], "error in (no error)"=w258, "fit to page width? (F)"=FALSE) -> ("report out"=w261:refnum<class "NI_report.lvclass">, "error out"=w262:errorcluster)  [unwired: 10 in]
      n133 = call-dynamic "Set Report Font.vi"("report in"=w261, "text options"=w296, "font settings"=w297, "error in (no error)"=w262) -> ("report out"=w246:refnum<class "NI_report.lvclass">, "error out"=w245:errorcluster)  [unwired: 9 in, 1 out]
      n134 = disable-structure shown="Enabled" {
        disable-tunnel: [w312 w313] -> w249
        disable-tunnel: [w311 w314] -> w248
        disable-tunnel: w247 -> [w310 _]
        disable-tunnel: w246 -> [w309 w314]
        disable-tunnel: w245 -> [w308 w313]
        disable-tunnel: w244 -> [w303 _]
        frame Disabled {
          n135 = call-dynamic "New Report Page.vi"("report in"=w309, "error in (no error)"=w308) -> ("report out"=w306:refnum<class "NI_report.lvclass">, "error out"=w307:errorcluster)  [unwired: 12 in]
          n136 = call-poly <vilib>:"Append Image to Report.vi"("report in"=w306, "path or URL of image"=w303, "error in (no error)"=w307) -> ("report out"=w305:refnum<class "NI_report.lvclass">, "error out"=w304:errorcluster)  [unwired: 9 in, 2 out]
          n137 = call <vilib>:"Word Insert Object.vi"("report in"=w305, "file path"=w310, "error in (no error)"=w304) -> ("report out"=w311:refnum<class "NI_report.lvclass">, "error out"=w312:errorcluster)  [unwired: 11 in]
        }
        frame Enabled {
        }
      }
      n138 = local read "RefArr"() -> (w284:u32[])
      n139 = call <vilib>:"Word Set Page Numbering.vi"("report in"=w248, "position (footers)"=w287, "alignment (right)"=w286, "error in (no error)"=w249) -> ("report out"=w289:refnum<class "NI_report.lvclass">, "error out"=w288:errorcluster)  [unwired: 10 in]
      n140 = for {
        N: w241 -> [_]
        tunnel: w284 -> [w367]
        shift-right: [w357] -> w291
        shift-left: w288 -> [w371]
        shift-right: [w358] -> w290
        shift-left: w289 -> [w372]
        tunnel: w244 -> [w360]
        tunnel: w239 -> [w355]
        i -> [w365]
        (unwired) FALSE ("append on new line? (F)")
        n141 = Increment(x=w365) -> (x+1=w375:i32)
        n142 = Index Array(array=w367, index=w365) -> (element=w366:u32)
        n143 = control-ref of="Steps   p1"() -> (w369:refnum<vi>)
        n144 = Number To Decimal String(number=w375, width (-)=i16 2) -> (decimal integer string=w373:string)
        n145 = Type Cast(type=w369, x=w366) -> (*(type *) &x=w370:refnum<vi>)
        n146 = call-dynamic "New Report Page.vi"("report in"=w372, "error in (no error)"=w371) -> ("report out"=w363:refnum<class "NI_report.lvclass">, "error out"=w364:errorcluster)  [unwired: 12 in]
        n147 = Concatenate Strings("p.", w373) -> ()  [unwired: 1 out]
        n148 = call-poly <vilib>:"Append Image to Report.vi"("report in"=w363, "path or URL of image"=w360, "error in (no error)"=w364) -> ("report out"=w362:refnum<class "NI_report.lvclass">, "error out"=w361:errorcluster)  [unwired: 9 in, 2 out]
        n149 = call-dynamic "Append Control Image to Report.vi"("report in"=w362, "image file type (.jpg)"=enum16{".jpg", ".png"}.".png" ("image file type(.jpg)"), "ctrl reference"=w370, "error in (no error)"=w361) -> ("report out"=w359:refnum<class "NI_report.lvclass">, "error out"=w356:errorcluster)  [unwired: 8 in, 2 out]
        n150 = call <vilib>:"Word Format Picture.vi"("report in"=w359, "height (-1)"=w355, "error in (no error)"=w356) -> ("report out"=w358:refnum<class "NI_report.lvclass">, "error out"=w357:errorcluster)  [unwired: 11 in]
      }
      n151 = call <vilib>:"Clear Errors.vi"("error in (no error)"=w291) -> ("error out"=w240:errorcluster)  [unwired: 5 in, 1 out]
      n152 = call-poly <vilib>:"Append Report Text.vi"("report in"=w290, "append on new line? (F)"=TRUE, "error in (no error)"=w240) -> ("report out"=w269:refnum<class "NI_report.lvclass">, "error out"=w268:errorcluster)  [unwired: 9 in, 2 out]
      n153 = call-dynamic "Save Report to File.vi"("report in"=w269, "report file path"="Report Folder", "error in (no error)"=w268) -> ("error out"=w242:errorcluster)  [unwired: 11 in, 1 out]
      n154 = call <vilib>:"Simple Error Handler.vi"("error in (no error)"=w242) -> ("error out"=w298:errorcluster)  [unwired: 4 in, 4 out]
      "path out" <- "Report Folder"
    }
  }
  "error out" <- "error in (no error)"
